vi "ConvertToXML.vi"(7 "InputTag":string="MeasurementResults", 8 "error in (no error)":errorcluster, 10 "DataInput":string[][](array[string]), 11 "DOM document in":refnum<k20>) -> (0 "error out":errorcluster, 2 "XML":string, 3 "DOM document out":refnum<k20>)   [LabVIEW 2013, in "main.lvlib"]
uses:
  main.lvlib
  <vilib>/xml/Close Reference(Node).vi
  <resource>/objmgr/DOMUserDefRef.rc
  <vilib>/xml/NI_XML.lvlib
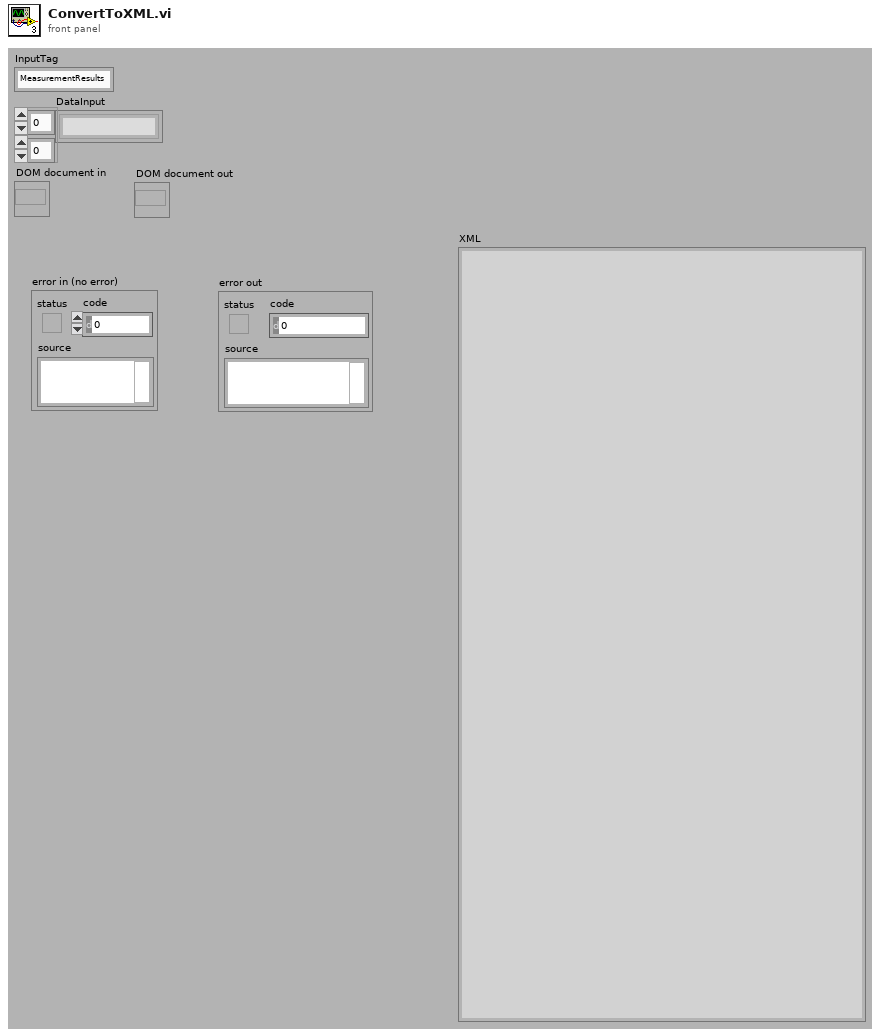
[diagram p1: front panel]
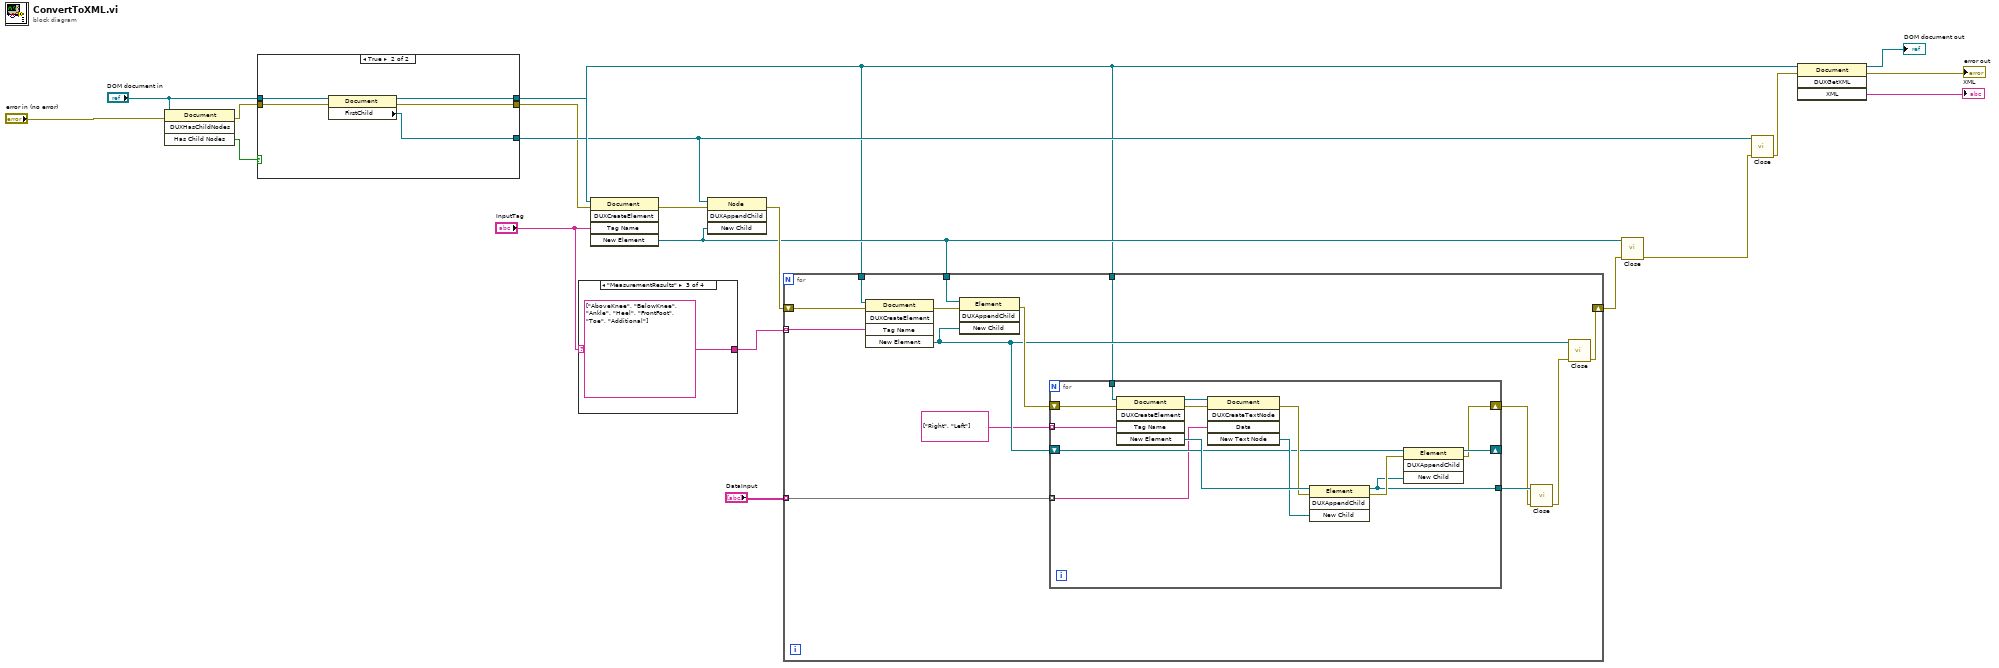
[diagram p0: block diagram]
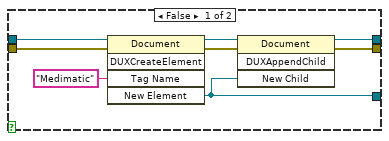
[diagram p2: hidden frame]
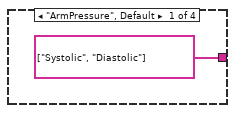
[diagram p3: hidden frame]
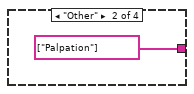
[diagram p4: hidden frame]
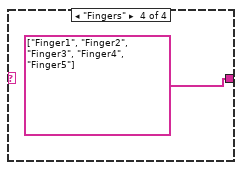
[diagram p5: hidden frame]
diagram:
  n1 = invoke class="Document" method="DUXHasChildNodes"(reference="DOM document in", error in="error in (no error)") -> (error out=w2:errorcluster, "Has Child Nodes"=w1:bool)  [unwired: 2 in, 2 out]
  n2 = case shown="True" w1 {
    tunnel: [w24 w29] -> w16
    tunnel: [w23 w28] -> w15
    tunnel: [w22 w30] -> w14
    tunnel: w2 -> [w21 w31]
    tunnel: "DOM document in" -> [w20 w32]
    frame False {
      n3 = invoke class="Document" method="DUXCreateElement"(reference=w20, error in=w21, "Tag Name"="Medimatic") -> (reference out=w27:refnum<k20>, error out=w26:errorcluster, "New Element"=w23:refnum<k20>)  [unwired: 2 in, 2 out]
      n4 = invoke class="Document" method="DUXAppendChild"(reference=w27, error in=w26, "New Child"=w23) -> (reference out=w24:refnum<k20>, error out=w22:errorcluster)  [unwired: 1 in, 2 out]
    }
    frame True {
      n5 = property class="Document"(reference=w32, error in=w31) -> (reference out=w29:refnum<k20>, error out=w30:errorcluster, "FirstChild"=w28:refnum<k20>)
    }
  }
  n6 = case shown="\"MeasurementResults\"" "InputTag" {
    tunnel: [string[] ["Systolic", "Diastolic"] string[] ["Palpation"] string[] ["AboveKnee", "BelowKnee", "Ankle", "Heel", "FrontFoot", "Toe", "Additional"] string[] ["Finger1", "Finger2", "Finger3", "Finger4", "Finger5"]] -> w18
    frame "ArmPressure", Default {
    }
    frame "Other" {
    }
    frame "MeasurementResults" {
    }
    frame "Fingers" {
    }
  }
  n7 = invoke class="Document" method="DUXCreateElement"(reference=w16, error in=w14, "Tag Name"="InputTag") -> (error out=w13:errorcluster, "New Element"=w9:refnum<k20>)  [unwired: 2 in, 3 out]
  n8 = invoke class="Node" method="DUXAppendChild"(reference=w15, error in=w13, "New Child"=w9) -> (error out=w12:errorcluster)  [unwired: 1 in, 3 out]
  n9 = for {
    tunnel: w9 -> [w44]
    tunnel: "DOM document in" -> [w43]
    tunnel: "DOM document in" -> [w42]
    shift-right: [w40] -> w11
    shift-left: w12 -> [w41]
    tunnel: w18 -> [w38] mode=indexing
    tunnel: "DataInput" -> [w37] mode=indexing
    n10 = invoke class="Document" method="DUXCreateElement"(reference=w43, error in=w41, "Tag Name"=w38) -> (error out=w50:errorcluster, "New Element"=w46:refnum<k20>)  [unwired: 2 in, 3 out]
    n11 = invoke class="Element" method="DUXAppendChild"(reference=w44, error in=w50, "New Child"=w46) -> (error out=w47:errorcluster)  [unwired: 1 in, 3 out]
    n12 = for {
      shift-right: [w55] -> w48
      shift-left: w47 -> [w57]
      shift-right: [w59] -> _
      shift-left: w46 -> [w56]
      tunnel: w42 -> [w54]
      tunnel: [w53] -> w49
      tunnel: string[] ["Right", "Left"] -> [w52] mode=indexing
      tunnel: w37 -> [w51] mode=indexing
      n13 = invoke class="Document" method="DUXCreateElement"(reference=w54, error in=w57, "Tag Name"=w52) -> (reference out=w64:refnum<k20>, error out=w63:errorcluster, "New Element"=w62:refnum<k20>)  [unwired: 2 in, 2 out]
      n14 = invoke class="Document" method="DUXCreateTextNode"(reference=w64, error in=w63, "Data"=w51) -> (error out=w61:errorcluster, "New Text Node"=w58:refnum<k20>)  [unwired: 2 in, 3 out]
      n15 = invoke class="Element" method="DUXAppendChild"(reference=w62, error in=w61, "New Child"=w58) -> (reference out=w53:refnum<k20>, error out=w60:errorcluster)  [unwired: 1 in, 2 out]
      n16 = invoke class="Element" method="DUXAppendChild"(reference=w56, error in=w60, "New Child"=w53) -> (reference out=w59:refnum<k20>, error out=w55:errorcluster)  [unwired: 1 in, 2 out]
    }
    n17 = call-poly <vilib>:"Close.vi"("error in (no error)"=w48, "node"=w49) -> ("error out"=w45:errorcluster)  [unwired: 7 in]
    n18 = call-poly <vilib>:"Close.vi"("error in (no error)"=w45, "node"=w46) -> ("error out"=w40:errorcluster)  [unwired: 7 in]
  }
  n19 = call-poly <vilib>:"Close.vi"("error in (no error)"=w11, "node"=w9) -> ("error out"=w10:errorcluster)  [unwired: 7 in]
  n20 = call-poly <vilib>:"Close.vi"("error in (no error)"=w10, "node"=w15) -> ("error out"=w17:errorcluster)  [unwired: 7 in]
  n21 = invoke class="Document" method="DUXGetXML"(reference="DOM document in", error in=w17) -> (reference out=→"DOM document out":refnum<k20>, error out=→"error out":errorcluster, "XML"=→"XML":string)  [unwired: 2 in, 1 out]
